vi "TestCase_Init.vi"(7 "GUID (\"\")":string, 8 "error in (no error)":errorcluster, 10 "methodName (\"runTest\")":string="runTest", 11 "TestCase in":refnum<class "TestCase.lvclass">) -> (0 "error out":errorcluster, 3 "TestCase out":refnum<class "TestCase.lvclass">)   [LabVIEW 2013, in "TestCase.lvclass"]
doc: "Initialize a TestCase object with methodName. methodName is the test method VI name (without .vi extension).\n\nThis VI should be called whenever a new TestCase object is needed such as during TestSuite.New method calls."
uses:
  TestCase.lvclass
  TestCase.lvclass/TestCase.ctl
  Libraries/VITesterUtilities.lvlib
panel:
  # "JKI VI Tester for LabVIEW\nhttp://jkisoft.com/vi-tester\nCopyright (C) 2007-2009, JKI <info@jkisoft.com>\nALL RIGHTS RESERVED"
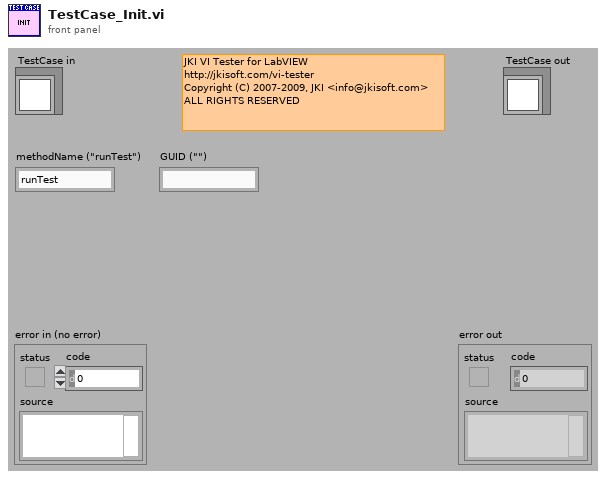
[diagram p1: front panel]
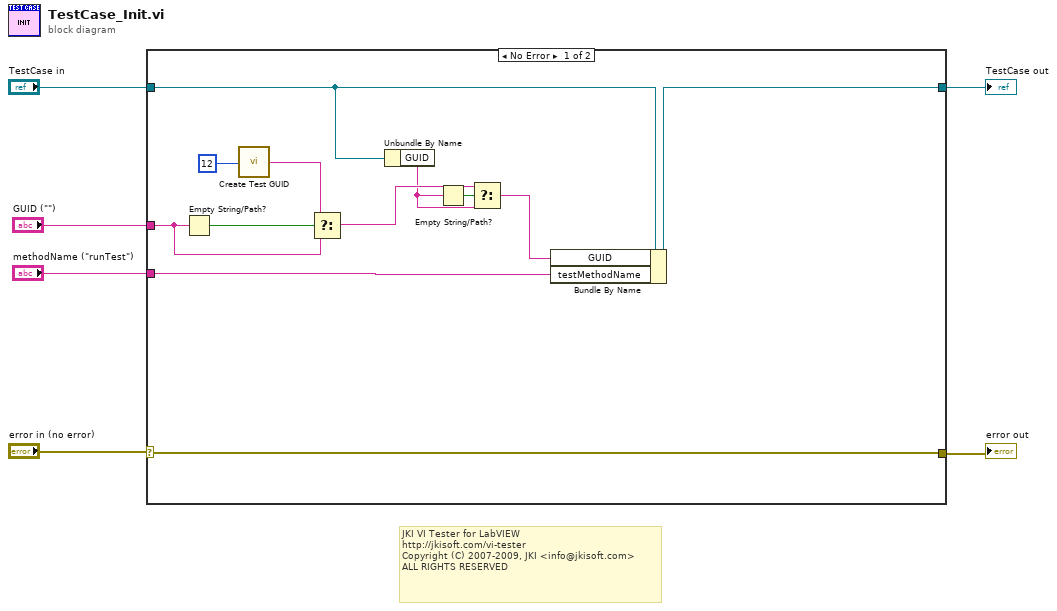
[diagram p0: block diagram]
diagram:
  # "JKI VI Tester for LabVIEW\nhttp://jkisoft.com/vi-tester\nCopyright (C) 2007-2009, JKI <info@jkisoft.com>\nALL RIGHTS RESERVED"
  n1 = case shown="No Error" "error in (no error)" {
    selector: "error in (no error)" -> [w16 w19]
    tunnel: "TestCase in" -> [w13 w20]
    tunnel: [w18 w20] -> w5
    tunnel: [w16 w19] -> w3
    tunnel: "methodName (\"runTest\")" -> [w17 _]
    tunnel: "GUID (\"\")" -> [w14 _]
    frame No Error {
      n2 = Empty String/Path?(string/path=w14) -> (empty?=w15:bool)
      n3 = call "Create Test GUID.vi"("length"=12) -> ("random data"=w7:string)  [unwired: 4 in]
      n4 = Select(t=w7, s=w15, f=w14) -> (s? t:f=w11:string)
      n5 = Unbundle By Name(w13) -> ("GUID"=w10:string)
      n6 = Empty String/Path?(string/path=w10) -> (empty?=w12:bool)
      n7 = Select(t=w11, s=w12, f=w10) -> (s? t:f=w9:string)
      n8 = Bundle By Name(cluster=w13, "GUID"=w9, "testMethodName"=w17) -> (w18:refnum<class "TestCase.lvclass">)
    }
    frame Error {
    }
  }
  "TestCase out" <- w5
  "error out" <- w3
